vi "writeFromeQueue.vi"(8 "queue":refnum<queue>, 11 "Cluster":T2) -> (0 "output cluster":T1, 2 "Data Write":string, 3 "GCODE WAIT   2":i32)   [LabVIEW 2017]
uses:
  mWorkToolkit/libSerial/stateSerialUltra.ctl
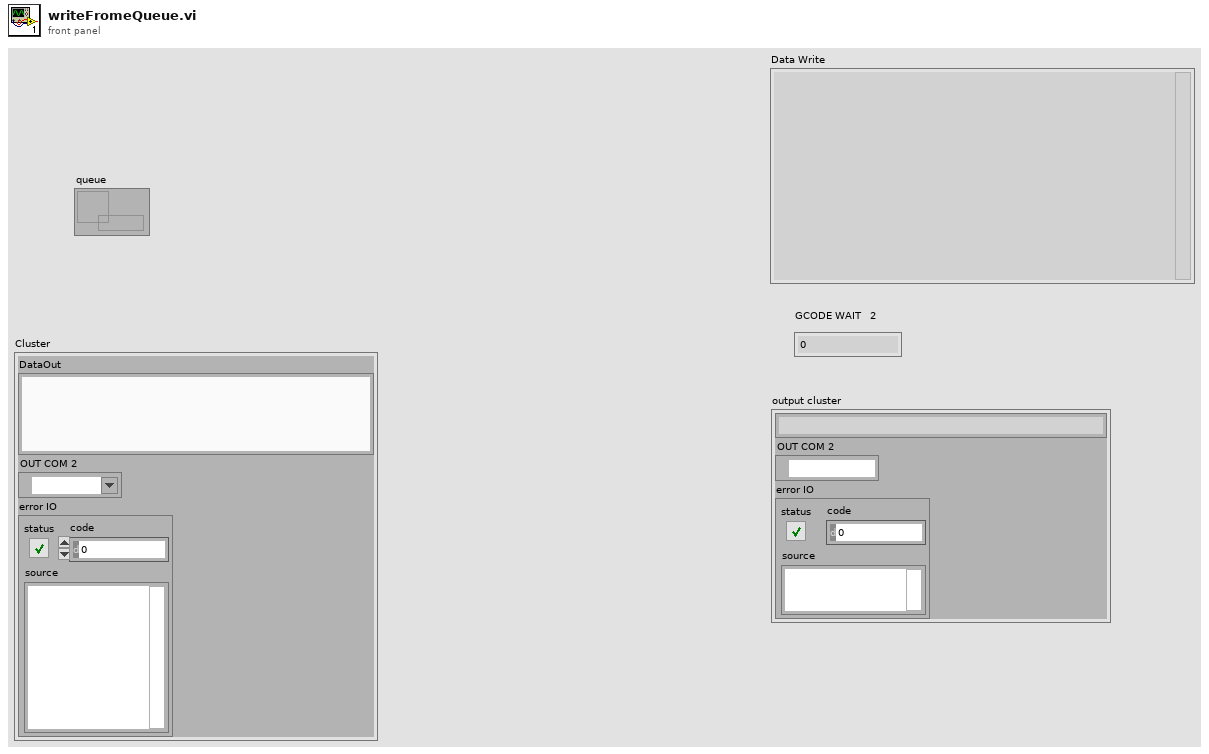
[diagram p1: front panel]
types:
  T1 = cluster{string, "OUT COM 2":refnum<visa-resource-name>, "error IO":errorcluster}
  T2 = cluster{"DataOut":string, "OUT COM 2":refnum<visa-resource-name>, "error IO":errorcluster}
  T3 = typedef "stateSerialUltra.ctl" = enum16{"findCOM", "Init", "CheckConnect", "Read", "Write", "exit"}
  T4 = cluster{"DataOut":string, "OUT COM 2":refnum<visa-resource-name>, "error out":errorcluster}
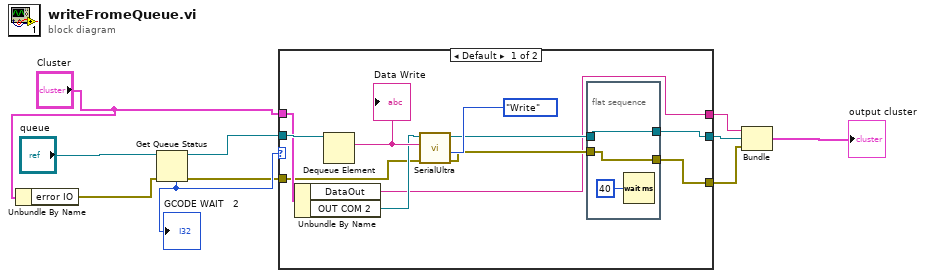
[diagram p0: block diagram]
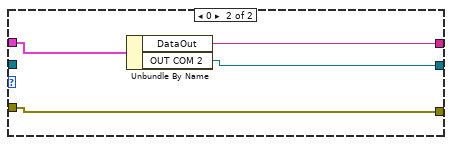
[diagram p2: hidden frame]
diagram:
  n1 = Unbundle By Name("Cluster") -> ("error IO"=w2:errorcluster)
  n2 = Get Queue Status(queue="queue", error in (no error)=w2) -> (queue out=w7:refnum<queue>, error out=w3:errorcluster, # elements in queue=w8:i32)  [unwired: 1 in, 5 out]
  "GCODE WAIT   2" <- w8
  n3 = case shown="Default" w8 {
    tunnel: [w15 w26] -> w9
    tunnel: [w14 w27] -> w10
    tunnel: w7 -> [w19 _]
    tunnel: "Cluster" -> [w18 w28]
    tunnel: w3 -> [w12 w26]
    tunnel: [w11 w25] -> w1
    frame Default {
      n4 = Unbundle By Name(w18) -> ("DataOut"=w11:string, "OUT COM 2"=w17:refnum<visa-resource-name>)
      n5 = Dequeue Element(queue=w19) -> (element=w21:string)  [unwired: 2 in, 3 out]
      "Data Write" <- w21
      n6 = call "SerialUltra.vi"("error in"=w12, "State"=stateSerialUltra."Write", "Data Write"=w21, "IN COM"=w17) -> ("error out"=w16:errorcluster, "OUT COM 2"=w13:refnum<visa-resource-name>)  [unwired: 3 in, 3 out]
      n7 = flat-sequence {
        tunnel: w16 -> [w24]
        tunnel: [w24] -> w15
        tunnel: [w22] -> w14
        tunnel: w13 -> [w22]
        frame #0 {
          n8 = Wait (ms)(milliseconds to wait=u32 40) -> ()  [unwired: 1 out]
        }
      }
    }
    frame 0 {
      n9 = Unbundle By Name(w28) -> ("DataOut"=w25:string, "OUT COM 2"=w27:refnum<visa-resource-name>)
    }
  }
  n10 = Bundle("DataOut"=w1, "OUT COM 2"=w10, "error out"=w9) -> (→"output cluster":T4)  [unwired: 1 in]
